vi "Open Wave File.vi"(9 "open original files":bool, 11 "start path":path) -> (0 "cancelled":bool, 1 "sound format":T1, 2 "wave data":i16[](array[numeric]), 3 "wave file path out":path)   [LabVIEW 2017]
uses:
  <vilib>/addons/Sound and Vibration/Order Analysis/Example Support/Demo VI/Start-Up Kit/File Access/Sound Format+.ctl
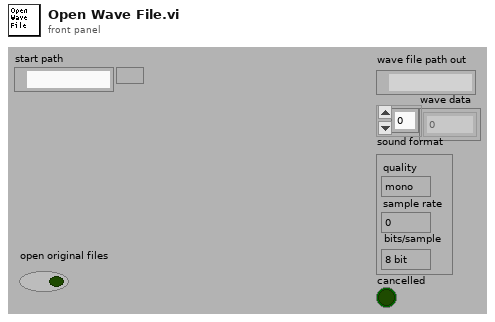
[diagram p1: front panel]
types:
  T1 = typedef "Sound Format+.ctl" = cluster{"quality":enum16{"mono", "stereo"}, "sample rate":u32, "bits/sample":enum16{"8 bit", "16 bit"}}
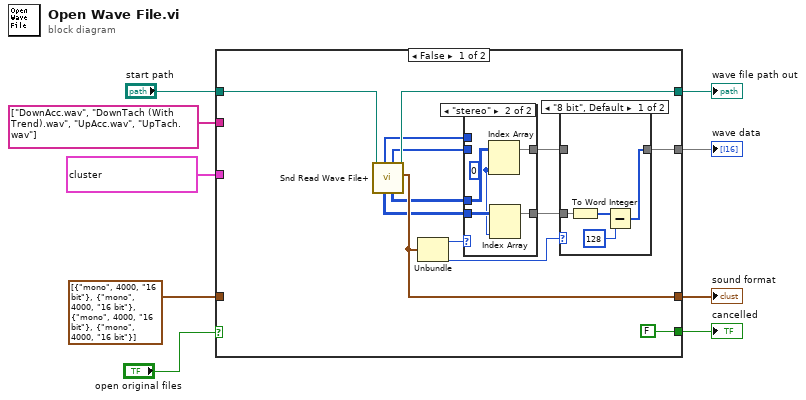
[diagram p0: block diagram]
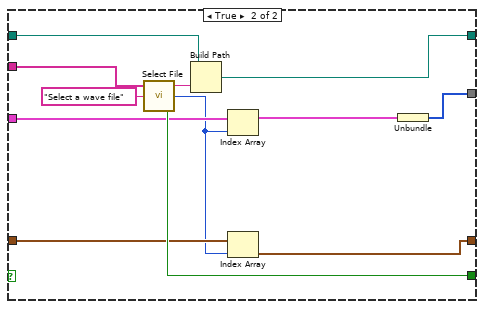
[diagram p4: hidden frame]
diagram:
  n1 = case shown="False" "open original files" {
    tunnel: "start path" -> [w11 w45]
    tunnel: [w22 w44] -> w7
    tunnel: [FALSE ("canceled") w43] -> w6
    tunnel: [w13 w37] -> w5
    tunnel: [w21 w39] -> w4
    tunnel: cluster{i16[]}[] [{array[68608 elements]}, {array[68608 elements]}, {array[53248 elements]}, {array[53248 elements]}] ("Wave File Datas") -> [_ w42]
    tunnel: T1[] [{"quality"=enum."mono", "sample rate"=4000, "bits/sample"=enum."16 bit"}, {"quality"=enum."mono", "sample rate"=4000, "bits/sample"=enum."16 bit"}, {"quality"=enum."mono", "sample rate"=4000, "bits/sample"=enum."16 bit"}, {"quality"=enum."mono", "sample rate"=4000, "bits/sample"=enum."16 bit"}] ("sound format") -> [_ w41]
    tunnel: string[] ["DownAcc.wav", "DownTach (With Trend).wav", "UpAcc.wav", "UpTach.wav"] ("file names") -> [_ w36]
    frame False {
      n2 = call <vilib>:"Snd Read Wave File+.vi"("wave file path"=w11) -> ("sound format"=w21:T1, "wave file path out"=w22:path, "stereo 16-bit"=w17:i16[][], "mono 16-bit"=w18:i16[], "stereo 8-bit"=w16:u8[][], "mono 8-bit"=w19:u8[])  [unwired: 4 in, 1 out]
      n3 = Unbundle(w21) -> ("quality"=w20:enum16{"mono", "stereo"}, "bits/sample"=w14:enum16{"8 bit", "16 bit"})  [unwired: 1 out]
      n4 = case shown="\"stereo\"" w20 {
        tunnel: w19 -> [w28 _]
        tunnel: w18 -> [w29 _]
        tunnel: w17 -> [_ w34]
        tunnel: w16 -> [_ w33]
        tunnel: [w29 w32] -> w15
        tunnel: [w28 w31] -> w12
        frame "mono", Default {
        }
        frame "stereo" {
          w30 = 0 ("Disabled Index (col)")
          n5 = Index Array(array=w34, index (col)=w30) -> (element=w32:i16[])  [unwired: 1 in]
          n6 = Index Array(array=w33, index (col)=w30) -> (element=w31:u8[])  [unwired: 1 in]
        }
      }
      n7 = case shown="\"8 bit\", Default" w14 {
        tunnel: w15 -> [_ w27]
        tunnel: [w25 w27] -> w13
        tunnel: w12 -> [w26 _]
        frame "8 bit", Default {
          n8 = To Word Integer(number=w26) -> (16bit integer=w24:i16[])
          n9 = Subtract(x=w24, y=i16 128) -> (x-y=w25:i16[])
        }
        frame "16 bit" {
        }
      }
    }
    frame True {
      n10 = call <vilib>:"Select File.vi"("prompt"="Select a wave file", "file names"=w36) -> ("canceled"=w43:bool, "index"=w40:i32, "file name"=w46:string)  [unwired: 1 in]
      n11 = Build Path(base path=w45, name or relative path=w46) -> (appended path=w44:path)
      n12 = Index Array(array=w42, index=w40) -> (element=w38:cluster{i16[]})
      n13 = Index Array(array=w41, index=w40) -> (element=w39:T1)
      n14 = Unbundle(w38) -> (w37:i16[])
    }
  }
  "wave file path out" <- w7
  "cancelled" <- w6
  "wave data" <- w5
  "sound format" <- w4
